vi "LJM_eStreamStop.vi"(0 "Handle In":i32, 11 "error in":errorcluster) -> (4 "Handle Out":i32, 15 "error out":errorcluster)   [LabVIEW 2025]
uses:
  labjackm.dll
panel:
  # "Calls eStreamStop even if error in is true."
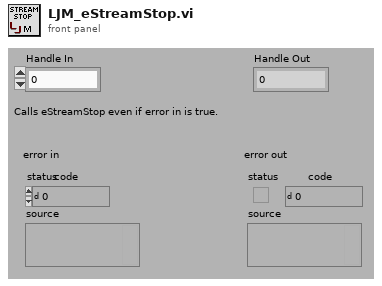
[diagram p1: front panel]
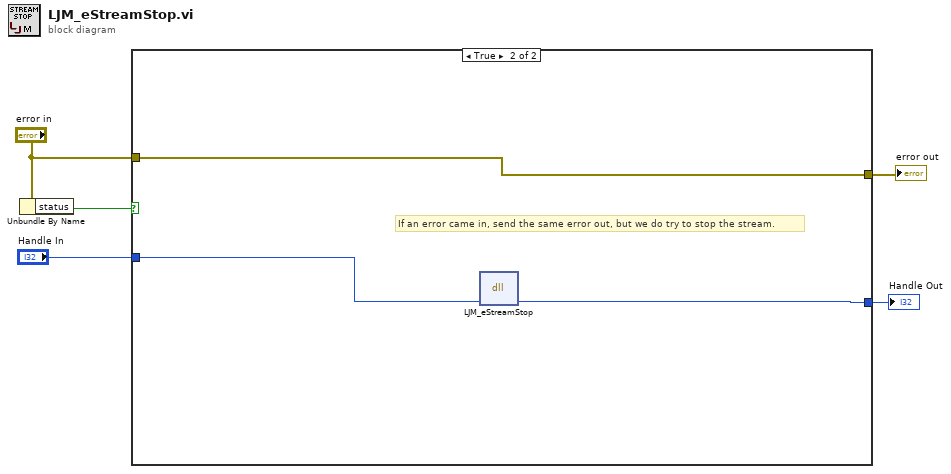
[diagram p0: block diagram]
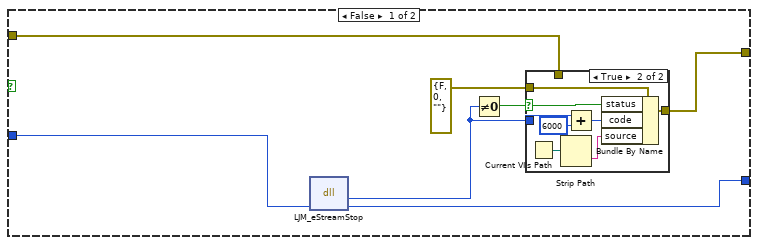
[diagram p2: hidden frame]
diagram:
  n1 = Unbundle By Name("error in") -> ("status"=w5:bool)
  n2 = case shown="True" w5 {
    tunnel: "error in" -> [w8 w24]
    tunnel: [w9 w24] -> w3
    tunnel: [w7 w22] -> w2
    tunnel: "Handle In" -> [w6 w23]
    frame False {
      n3 = dll-call lib="labjackm.dll" fn="LJM_eStreamStop"("Handle"=w6) -> (w12:i32, "Handle"=w7:i32)  [unwired: 3 in, 2 out]
      n4 = Not Equal To 0?(x=w12) -> (x != 0?=w11:bool)
      n5 = case shown="True" w11 {
        selector: w11 -> [_ w20]
        tunnel: [w13 w21] -> w9
        tunnel: errorcluster {"status"=FALSE, "code"=0, "source"=""} ("error IO") -> [_ w19]
        tunnel: w12 -> [_ w15]
        tunnel: w8 -> [w13 _]
        frame False {
        }
        frame True {
          n6 = Current VI's Path() -> (path=w17:path)
          n7 = Strip Path(path=w17) -> (name=w18:string)  [unwired: 1 out]
          n8 = Add(x=w15, y=6000) -> (x+y=w16:i32)
          n9 = Bundle By Name(cluster=w19, "status"=w20, "code"=w16, "source"=w18) -> (w21:errorcluster)
        }
      }
    }
    frame True {
      # "If an error came in, send the same error out, but we do try to stop the stream."
      n10 = dll-call lib="labjackm.dll" fn="LJM_eStreamStop"("Handle"=w23) -> ("Handle"=w22:i32)  [unwired: 4 in, 2 out]
    }
  }
  "error out" <- w3
  "Handle Out" <- w2
